vi "Toggle DO Line.vi"(6 "Simulate":bool, 7 "ToggleWaitIntv (ms)":u32=250, 8 "error in":errorcluster, 9 "timeout":dbl=10.0 format="%0.2f", 10 "InitialState":bool=TRUE, 11 "DO-Line Ref":refnum<k21>) -> (0 "error out":errorcluster, 3 "DO-Line Ref out":refnum<k21>)   [LabVIEW 2017]
doc: "Developed by Kevin Thompson\nThompson Engineering, LLC\nkevin@thompsonengineering.net"
uses:
  <vilib>/DAQmx/write.llb/DAQmx Write (Digital Bool 1Line 1Point).vi
  <vilib>/DAQmx/miscellaneous.llb/DAQmx Fill In Error Info.vi
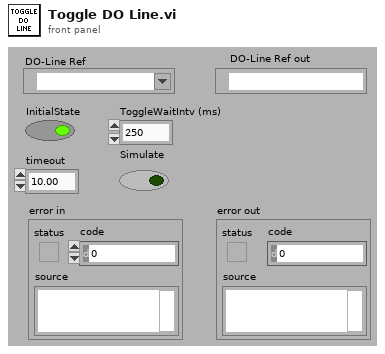
[diagram p1: front panel]
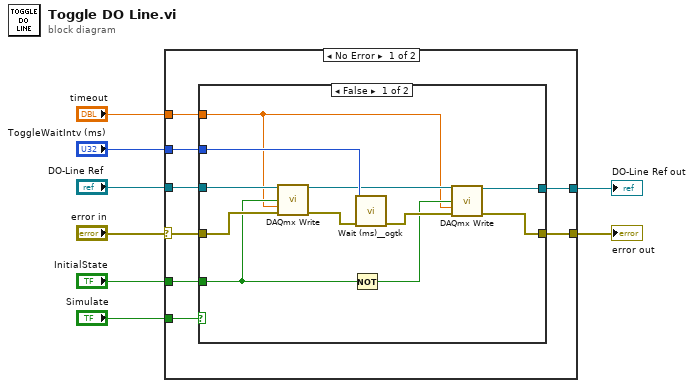
[diagram p0: block diagram]
diagram:
  n1 = case shown="No Error" "error in" {
    selector: "error in" -> [w9 w30]
    tunnel: [w16 w30] -> w8
    tunnel: "ToggleWaitIntv (ms)" -> [w15 _]
    tunnel: "DO-Line Ref" -> [w14 w31]
    tunnel: [w13 w31] -> w5
    tunnel: "InitialState" -> [w12 _]
    tunnel: "timeout" -> [w11 _]
    tunnel: "Simulate" -> [w10 _]
    frame No Error {
      n2 = case shown="False" w10 {
        tunnel: [w27 w28] -> w16
        tunnel: w9 -> [w26 w28]
        tunnel: w15 -> [w23 _]
        tunnel: w14 -> [w21 w29]
        tunnel: [w20 w29] -> w13
        tunnel: w12 -> [w19 _]
        tunnel: w11 -> [w17 _]
        frame False {
          n3 = call-poly <vilib>:"DAQmx Write.vi"("task/channels in"=w21, "data"=w19, "timeout"=w17, "error in"=w26) -> ("task out"=w22:refnum<k21>, "error out"=w24:errorcluster)  [unwired: 9 in, 1 out]
          n4 = Not(x=w19) -> (.not. x?=w18:bool)
          n5 = call <userlib>:"Wait (ms)__ogtk.vi"("error in (no error)"=w24, "milliseconds to wait"=w23) -> ("error out"=w25:errorcluster)  [unwired: 8 in, 1 out]
          n6 = call-poly <vilib>:"DAQmx Write.vi"("task/channels in"=w22, "data"=w18, "timeout"=w17, "error in"=w25) -> ("task out"=w20:refnum<k21>, "error out"=w27:errorcluster)  [unwired: 9 in, 1 out]
        }
        frame True {
        }
      }
    }
    frame Error {
    }
  }
  "error out" <- w8
  "DO-Line Ref out" <- w5
